vi "ProgressBar.TestLauncher.vi"() -> ()   [LabVIEW 2019, in "ProgressBar.lvclass"]
doc: "JKI State Machine Objects (SMO) 1.0.0.5\nJKI - JKI\nCopyright (c) 2016, JKI"
uses:
  ProgressBar.lvclass
  ProgressBar.lvclass/ProgressBar.ctl
  <vilib>/LabVIEW Open Source Project/Unicity/RandomStringGenerator/RandomStringGenerator.lvclass
panel:
  out "error out":errorcluster
  # "SMO Progress Bar Launcher"
  # "For instructions on how to use the JKI State Machine Objects, examples and video tutorials, visit:\nhttp://jki.net/state-machine-objects/\n\nJKI State Machine Objects™\nhttp://jki.net/state-machine-objects/\nCopyright (C) 2005-2015, JKI <info@jki.net>\nALL RIGHTS RESERVED"
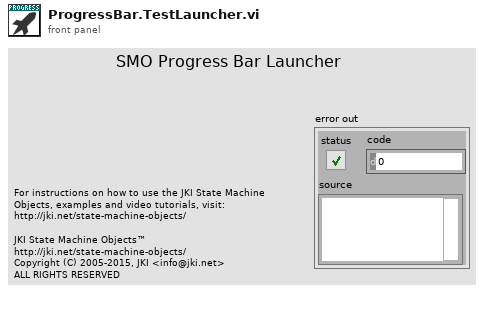
[diagram p1: front panel]
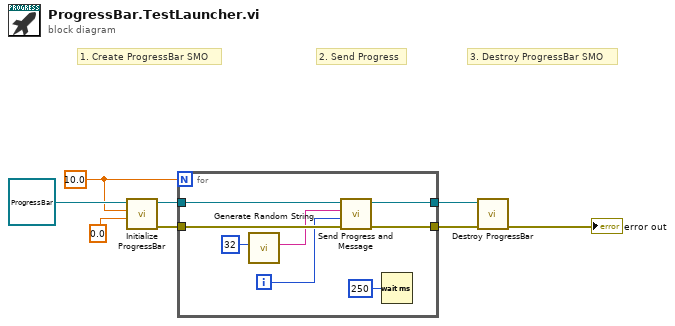
[diagram p0: block diagram]
diagram:
  w1 = 10.0 ("Config.Scale Max")
  # "3. Destroy ProgressBar SMO"
  # "2. Send Progress"
  # "1. Create ProgressBar SMO"
  n1 = call "Initialize ProgressBar.vi"("Scale Min"=0.0 ("Config.Scale Min"), "Scale Max"=w1, "ProgressBar in"=refnum<class "ProgressBar.lvclass"> refnum ("SMO.Template.lvclass")) -> ("error out"=w6:errorcluster, "ProgressBar out"=w5:refnum<class "ProgressBar.lvclass">)  [unwired: 7 in]
  n2 = for {
    N: w1 -> [_]
    tunnel: w5 -> [w15]
    tunnel: [w14] -> w4
    tunnel: w6 -> [w16]
    tunnel: [w13] -> w3
    i -> [w12]
    n3 = call <vilib>:"Generate Random String.vi"("String Length (32)"=u32 32) -> ("Random String"=w11:string)  [unwired: 10 in]
    n4 = call "Send Progress and Message.vi"("error in (no error)"=w16, "Progress"=w12, "Message"=w11, "ProgressBar in"=w15) -> ("error out"=w13:errorcluster, "ProgressBar out"=w14:refnum<class "ProgressBar.lvclass">)  [unwired: 6 in]
    n5 = Wait (ms)(milliseconds to wait=u32 250) -> ()  [unwired: 1 out]
  }
  n6 = call "Destroy ProgressBar.vi"("error in (no error)"=w3, "ProgressBar in"=w4) -> ("error out"=→"error out":errorcluster)  [unwired: 8 in, 1 out]
